vi "test_pid.vi"() -> ()   [LabVIEW 2019]
uses:
  <vilib>/addons/control/pid/pid.llb/PID (DBL).vi
  <vilib>/addons/control/pid/NI_PID_pid.lvlib
panel:
  in  "PID cfg":T1={"PID gains"={"proportional gain (Kc)"=0.002499999999999999, "integral time (Ti, min)"=0.0, "derivative time (Td, min)"=0.0}, "PID limits"={"output high"=0.07, "output low"=-0.07}, "dt_pid"=100} {"PID limits"."output low" format="%.3f"; "PID limits"."output high" format="%.3f"; "PID gains"."derivative time (Td, min)" format="%.4f"; "PID gains"."integral time (Ti, min)" format="%.4f"; "PID gains"."proportional gain (Kc)" format="%.4f"}
  in  "reinitialize? (F)":bool
  out "Waveform Chart":dbl(graph)
  in  "stop":bool
  in  "process variable":dbl(slide) scale=-50.0..42.0
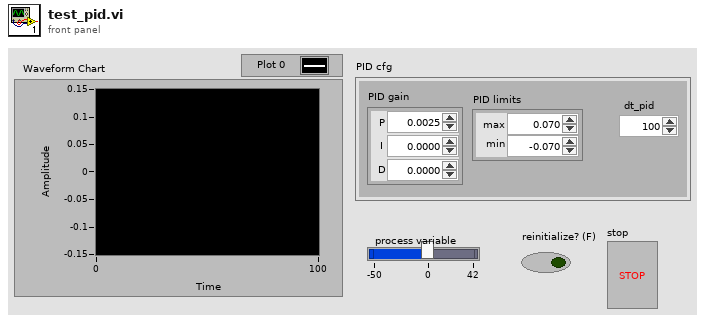
[diagram p1: front panel]
types:
  T1 = cluster{"PID gains":cluster{"proportional gain (Kc)":dbl, "integral time (Ti, min)":dbl, "derivative time (Td, min)":dbl}, "PID limits":cluster{"output high":dbl, "output low":dbl}, "dt_pid":u32}
  T2 = cluster{"proportional gain (Kc)":dbl, "integral time (Ti, min)":dbl, "derivative time (Td, min)":dbl}
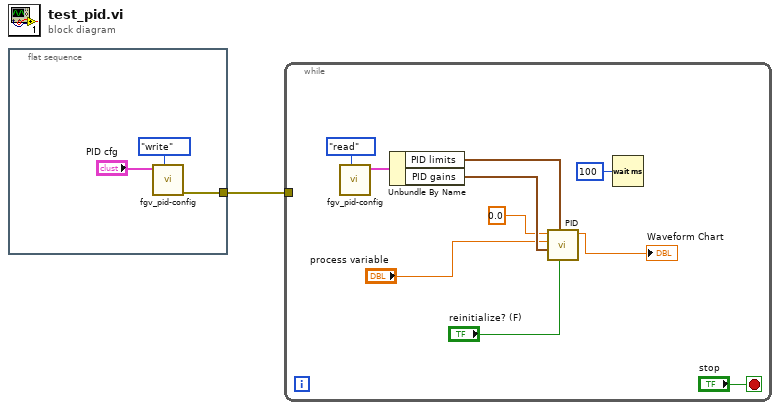
[diagram p0: block diagram]
diagram:
  n1 = flat-sequence {
    tunnel: [w3] -> w1
    frame #0 {
      n2 = call "fgv_pid-config.vi"("cmd"=enum16{"read", "write"}."write", "PID cfg"="PID cfg") -> ("error out"=w3:errorcluster)  [unwired: 8 in, 1 out]
    }
  }
  n3 = while {
    tunnel: w1 -> [_]
    stop <- "stop" stop-if-true
    n4 = call "fgv_pid-config.vi"("cmd"=enum16{"read", "write"}."read") -> ("PID cfg out"=w13:T1)  [unwired: 9 in, 1 out]
    n5 = Unbundle By Name(w13) -> ("PID limits"=w12:cluster{"output high":dbl, "output low":dbl}, "PID gains"=w11:T2)
    n6 = call-poly <vilib>:"PID.vi"("reinitialize? (F)"="reinitialize? (F)", "output range"=w12, "PID gains"=w11, "process variable"="process variable", "setpoint"=0.0) -> ("output"=→"Waveform Chart":dbl)  [unwired: 5 in, 1 out]
    n7 = Wait (ms)(milliseconds to wait=u32 100) -> ()  [unwired: 1 out]
  }
